vi "RandomLaser20-2.vi"() -> ()   [LabVIEW 2014]
uses:
  State-MainLoop.ctl
  <userlib>/_OpenG.lib/array/array.llb/Delete Elements from 2D Array (DBL)__ogtk.vi
panel:
  in  "Tab Control":T1(tab)
  out "Intensity Graph":dbl[][](graph)
  in  "Average":i32=1
  in  "Integration Time":i32=100
  out "Spectrum":T2(graph)
  in  "Custom Marker Colors":u32[](array[colorbox])=[9567230, 1187327, 3465]
  in  "Buffer Graph":i32=30
  in  "index (row)":i32
  in  "Select Light Source":u16(ring)
  out "Power Meter (W)":dbl=0.009689930499999999 format="%#_4p"
  out "Power Graph":dbl[](graph)
  in  "StepperMotor":bool
  out "Steps Chart":dbl(graph)
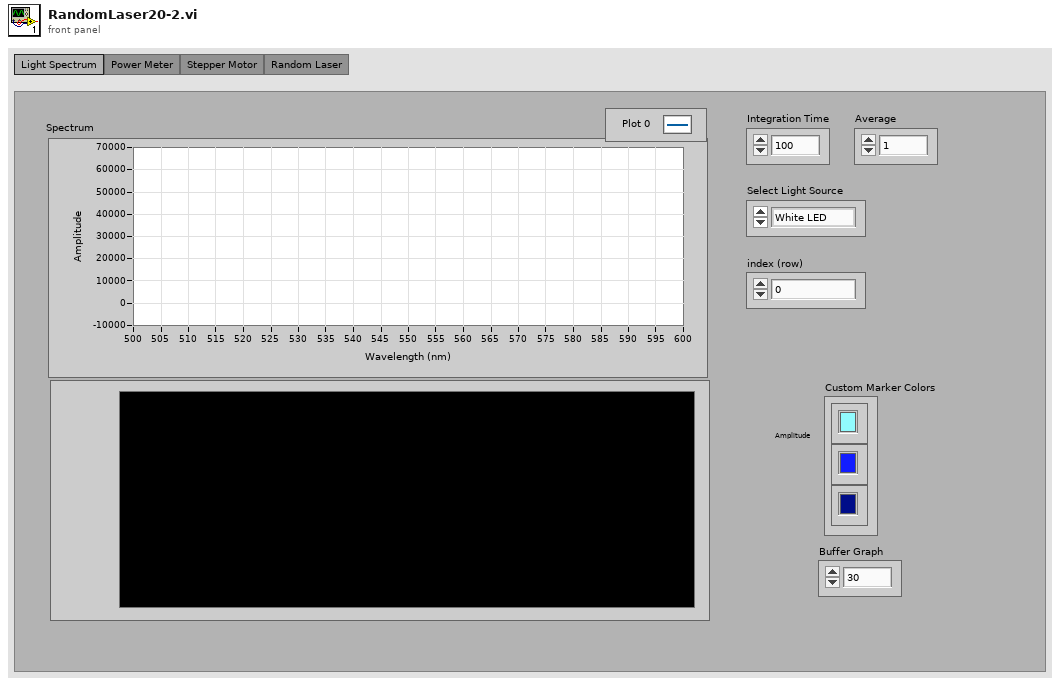
[diagram p1: front panel]
types:
  T1 = enum32{"Light Spectrum", "Power Meter", "Stepper Motor", "Random Laser"}
  T2 = cluster{"WL Values":dbl[], "Spectrum Values":dbl[]}
  T3 = typedef "State-MainLoop.ctl" = enum16{"Initialize", "Wait for Event", "Spectrum Graph", "Power Meter", "Stepper Motor", "Random Laser"}
  T4 = enum32{"Page Enabled", "Page Disabled", "Page Disabled & Grayed"}
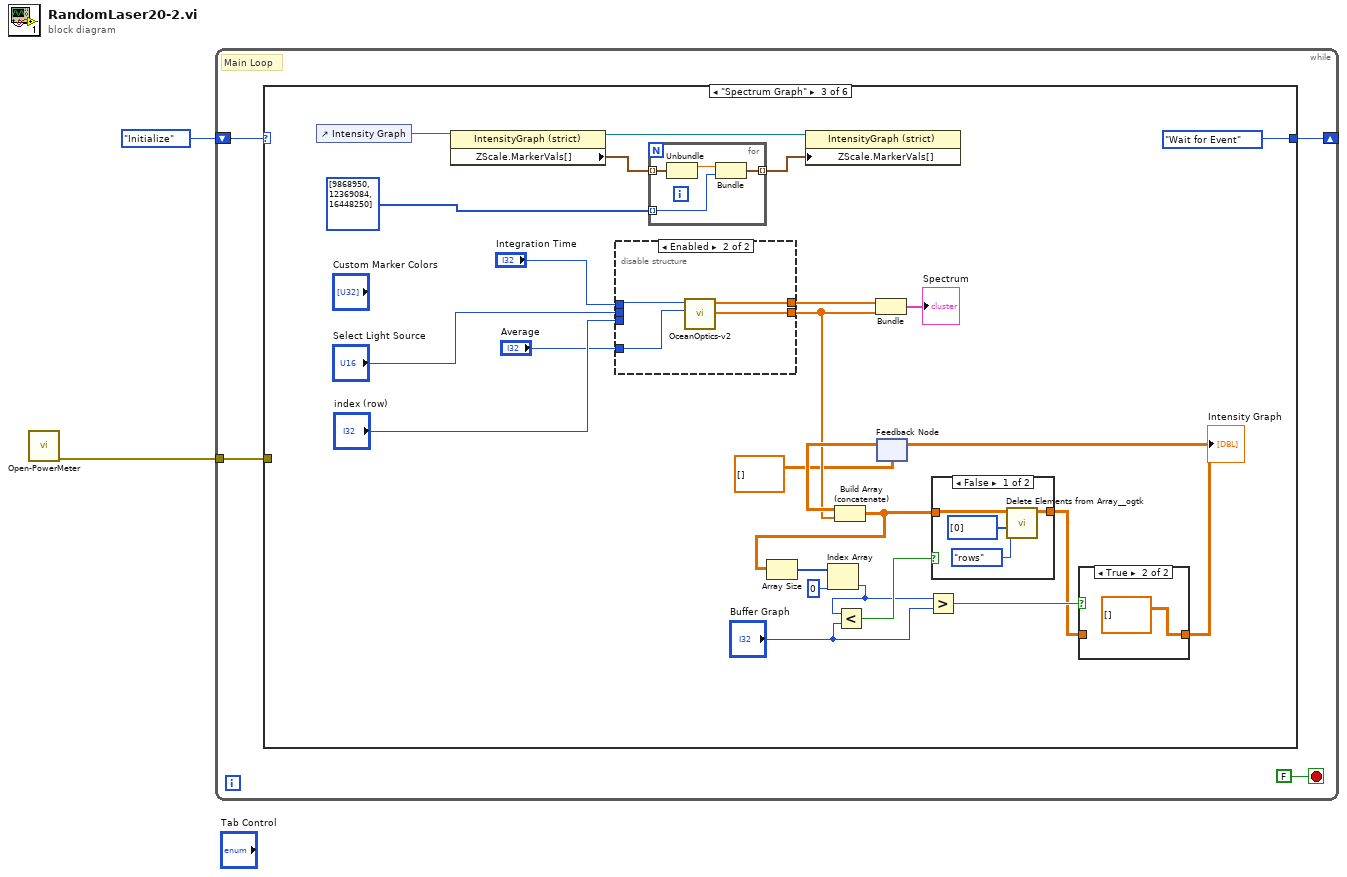
[diagram p0: block diagram]
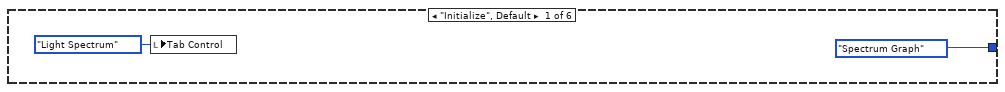
[diagram p2: hidden frame]
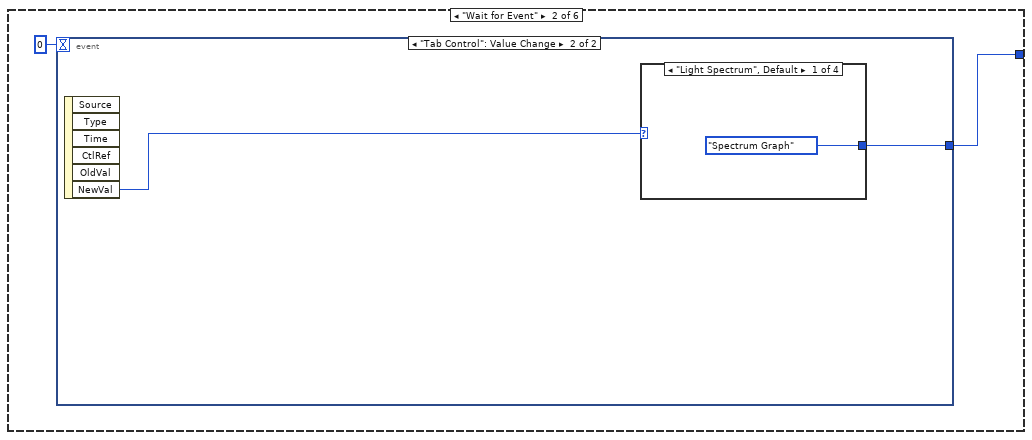
[diagram p3: hidden frame]
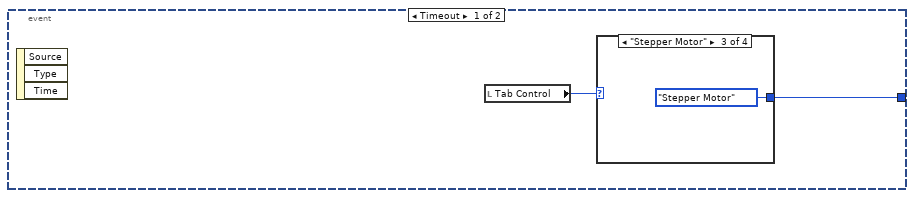
[diagram p4: hidden frame]
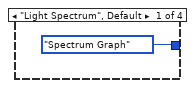
[diagram p5: hidden frame]
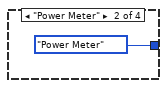
[diagram p6: hidden frame]
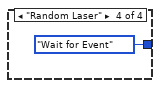
[diagram p7: hidden frame]
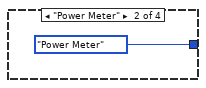
[diagram p8: hidden frame]
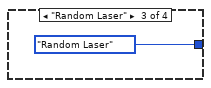
[diagram p9: hidden frame]
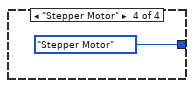
[diagram p10: hidden frame]
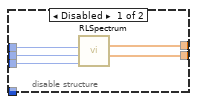
[diagram p11: hidden frame]
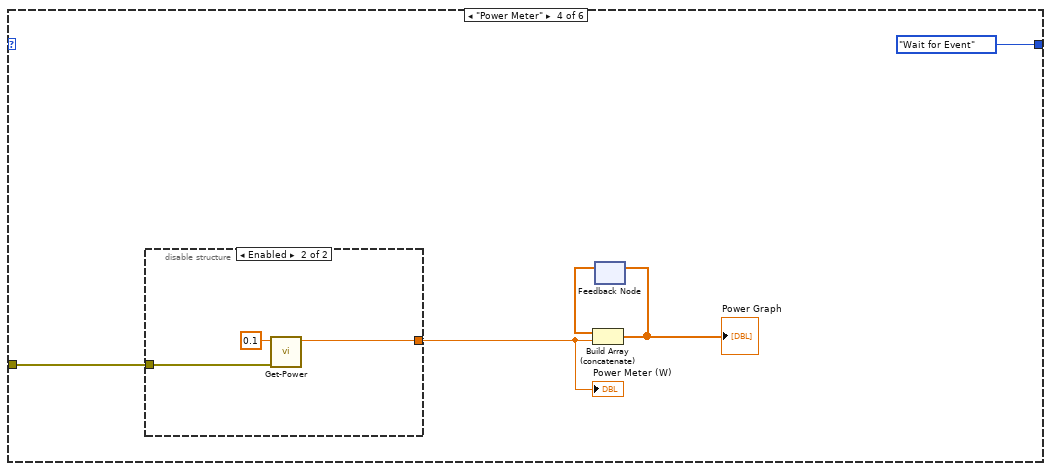
[diagram p14: hidden frame]
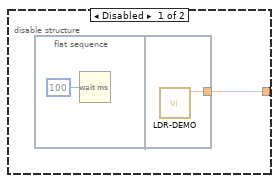
[diagram p15: hidden frame]
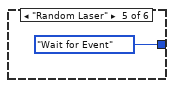
[diagram p16: hidden frame]
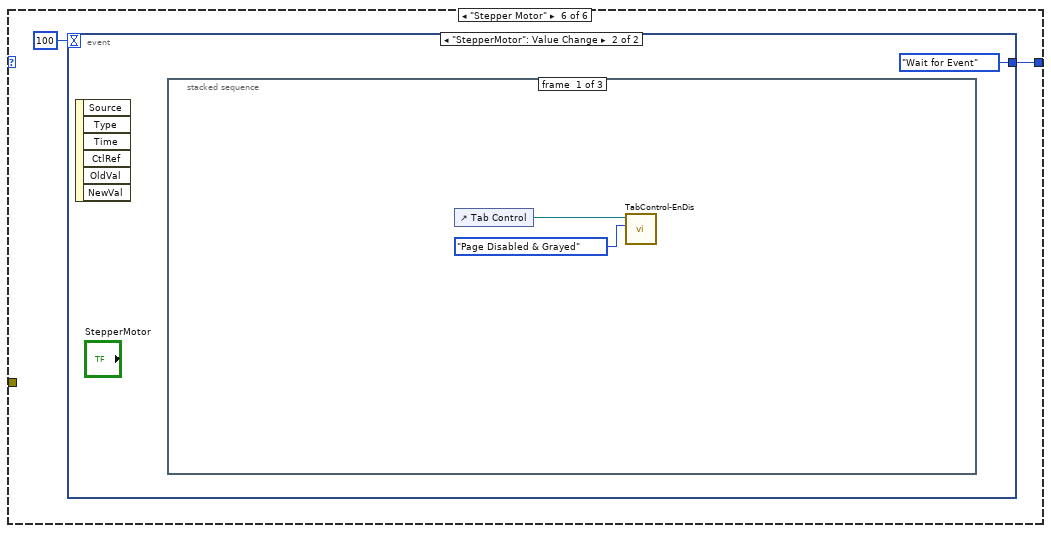
[diagram p17: hidden frame]
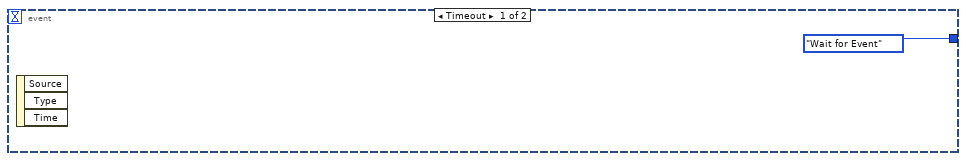
[diagram p18: hidden frame]
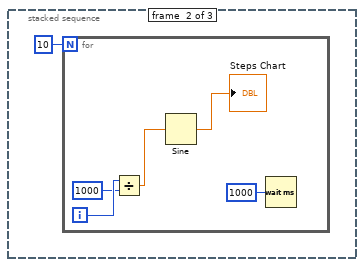
[diagram p19: hidden frame]
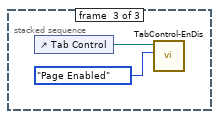
[diagram p20: hidden frame]
diagram:
  n1 = call "Open-PowerMeter.vi"() -> ("error out"=w1:errorcluster)  [unwired: 10 in, 1 out]
  n2 = while {
    shift-right: [w4] -> _
    shift-left: State-MainLoop."Initialize" -> [w5]
    tunnel: w1 -> [w3]
    stop <- FALSE stop-if-true
    # "Main Loop"
    n3 = case shown="\"Spectrum Graph\"" w5 {
      tunnel: [State-MainLoop."Spectrum Graph" w10 State-MainLoop."Wait for Event" State-MainLoop."Wait for Event" State-MainLoop."Wait for Event" w79] -> w4
      tunnel: w3 -> [_ _ _ w68 _ _]
      frame "Initialize", Default {
        n4 = local write "Tab Control"(T1."Light Spectrum" ("Tab Control")) -> ()
      }
      frame "Wait for Event" {
        n5 = event shown="[1] \"Tab Control\": Value Change" {
          selector: _ -> [_ _]
          dyn-events: _ -> [_ _]
          timeout: 0 -> [_ _]
          tunnel: [w12 w17] -> w10
          event Timeout {
            n6 = event-data() -> ()  [unwired: 1 in, 3 out]
            n7 = local read "Tab Control"() -> (w11:T1)
            n8 = case shown="\"Stepper Motor\"" w11 {
              tunnel: [State-MainLoop."Spectrum Graph" State-MainLoop."Power Meter" State-MainLoop."Stepper Motor" State-MainLoop."Wait for Event"] -> w12
              frame "Light Spectrum", Default {
              }
              frame "Power Meter" {
              }
              frame "Stepper Motor" {
              }
              frame "Random Laser" {
              }
            }
          }
          event "Tab Control": Value Change {
            n9 = event-data() -> ("NewVal"=w18:T1)  [unwired: 1 in, 5 out]
            n10 = case shown="\"Light Spectrum\", Default" w18 {
              tunnel: [State-MainLoop."Spectrum Graph" State-MainLoop."Power Meter" State-MainLoop."Random Laser" State-MainLoop."Stepper Motor"] -> w17
              frame "Light Spectrum", Default {
              }
              frame "Power Meter" {
              }
              frame "Random Laser" {
              }
              frame "Stepper Motor" {
              }
            }
          }
        }
      }
      frame "Spectrum Graph" {
        n11 = control-ref of="Intensity Graph"() -> (w37:refnum<vi>)
        n12 = property on="Property Node" class="IntensityGraph (strict)"(reference=w37) -> (reference out=w36:refnum<vi>, "ZScale.MarkerVals[]"=w43:cluster{dbl, u32}[])  [unwired: 1 in, 1 out]
        n13 = disable-structure shown="Enabled" {
          disable-tunnel: "Integration Time" -> [w51 w52]
          disable-tunnel: [w50 w54] -> w34
          disable-tunnel: [w49 w55] -> w33
          disable-tunnel: "index (row)" -> [w48 _]
          disable-tunnel: "Select Light Source" -> [w47 _]
          disable-tunnel: "Average" -> [_ w53]
          frame Disabled {
            n14 = call "RLSpectrum.vi"("index (row)"=w48, "Select Light Source"=w47, "Integration Time (ms)"=w51) -> ("Spectrum Values"=w50:dbl[], "WL Values"=w49:dbl[])  [unwired: 7 in]
          }
          frame Enabled {
            n15 = call "OceanOptics-v2.vi"("Average"=w53, "Integration Time (ms)"=w52) -> ("Y"=w54:dbl[], "X"=w55:dbl[])  [unwired: 7 in, 1 out]
          }
        }
        n16 = for {
          tunnel: w43 -> [w66] mode=indexing
          tunnel: u32[] [9868950, 12369084, 16448250] ("Custom Marker Colors") -> [w64] mode=indexing
          tunnel: [w63] -> w42 mode=indexing
          n17 = Unbundle(w66) -> (w65:dbl)  [unwired: 1 out]
          n18 = Bundle(w65, "Color Box"=w64) -> (w63:cluster{dbl, "Color Box":u32})  [unwired: 1 in]
        }
        n19 = property on="Property Node" class="IntensityGraph (strict)"(reference=w36, "ZScale.MarkerVals[]"=w42) -> ()  [unwired: 1 in, 2 out]
        n20 = Bundle("X"=w33, "Y"=w34) -> (→"Spectrum":cluster{"X":dbl[], "Y":dbl[]})  [unwired: 1 in]
        n21 = feedback #1(dbl[][] []) -> (w44:dbl[][])
        n22 = Build Array (concatenate)(w44, w34) -> (w41:dbl[][])
        n23 = Array Size(array=w41) -> (size(s)=w40:i32[])
        n24 = Index Array(array=w40, index=0) -> (element=w31:i32)
        n25 = Less?(x=w31, y="Buffer Graph") -> (x < y?=w38:bool)
        n26 = Greater?(x=w31, y="Buffer Graph") -> (0:w29:bool)
        n27 = case shown="False" w38 {
          tunnel: w41 -> [w61 w62]
          tunnel: [w60 w62] -> w28
          frame False {
            n28 = call-poly <userlib>:"Delete Elements from Array__ogtk.vi"("delete (rows or columns)"=enum16{"rows", "columns"}."rows", "indices"=i32[] [0], "array"=w61) -> ("array w/ subset deleted"=w60:dbl[][])  [unwired: 7 in, 1 out]
          }
          frame True {
          }
        }
        n29 = case shown="True" w29 {
          tunnel: w28 -> [w56 _]
          tunnel: [w56 dbl[][] []] -> w27
          frame False {
          }
          frame True {
          }
        }
        "Intensity Graph" <- w27
        n30 = feedback-in #1(w27) -> ()
      }
      frame "Power Meter" {
        n31 = disable-structure shown="Enabled" {
          disable-tunnel: w68 -> [_ w76]
          disable-tunnel: [w72 w75] -> w67
          frame Disabled {
            n32 = flat-sequence {
              tunnel: [w74] -> w72
              frame #0 {
                n33 = Wait (ms)(milliseconds to wait=u32 100) -> ()  [unwired: 1 out]
              }
              frame #1 {
                n34 = call "LDR-DEMO.vi"() -> ("Voltage"=w74:dbl)  [unwired: 10 in, 1 out]
              }
            }
          }
          frame Enabled {
            n35 = call "Get-Power.vi"("error in"=w76, "Average Time (0.0)"=0.1) -> ("Power"=w75:dbl)  [unwired: 8 in, 1 out]
          }
        }
        "Power Meter (W)" <- w67
        n36 = feedback #2() -> (w70:dbl[])  [unwired: 1 in]
        n37 = Build Array (concatenate)(w70, w67) -> (w69:dbl[])
        "Power Graph" <- w69
        n38 = feedback-in #2(w69) -> ()
      }
      frame "Random Laser" {
      }
      frame "Stepper Motor" {
        n39 = event shown="[1] \"StepperMotor\": Value Change" {
          selector: _ -> [_ _]
          dyn-events: _ -> [_ _]
          timeout: 100 -> [_ _]
          tunnel: [State-MainLoop."Wait for Event" State-MainLoop."Wait for Event"] -> w79
          event Timeout {
            n40 = event-data() -> ()  [unwired: 1 in, 3 out]
          }
          event "StepperMotor": Value Change {
            n41 = event-data() -> ()  [unwired: 1 in, 6 out]
            n42 = stacked-sequence {
              frame #0 {
                n43 = control-ref of="Tab Control"() -> (w83:refnum<vi>)
                n44 = call "TabControl-EnDis.vi"("Page Enabled State"=T4."Page Disabled & Grayed", "TabControl in"=w83) -> ()  [unwired: 9 in, 1 out]
              }
              frame #1 {
                n45 = for {
                  N: 10 -> [_]
                  i -> [w90]
                  n46 = Divide(x=w90, y=1000) -> (x/y=w88:dbl)
                  n47 = Sine(x=w88) -> (sin(x)=→"Steps Chart":dbl)
                  n48 = Wait (ms)(milliseconds to wait=u32 1000) -> ()  [unwired: 1 out]
                }
              }
              frame #2 {
                n49 = control-ref of="Tab Control"() -> (w91:refnum<vi>)
                n50 = call "TabControl-EnDis.vi"("Page Enabled State"=T4."Page Enabled", "TabControl in"=w91) -> ()  [unwired: 9 in, 1 out]
              }
            }
          }
        }
      }
    }
  }
